vi "REPORT_PACE_prepare_header_for_pdf.vi"(11 "REPORT_PACE_all_info":T1) -> (3 "report_header":string[][](array[string]))   [LabVIEW 2019]
uses:
  typedef/REPORT_PACE_all_info.ctl
  _misc/AULocalize/SubVIs/Get Localized Phrase Compact Interface 1D.vi
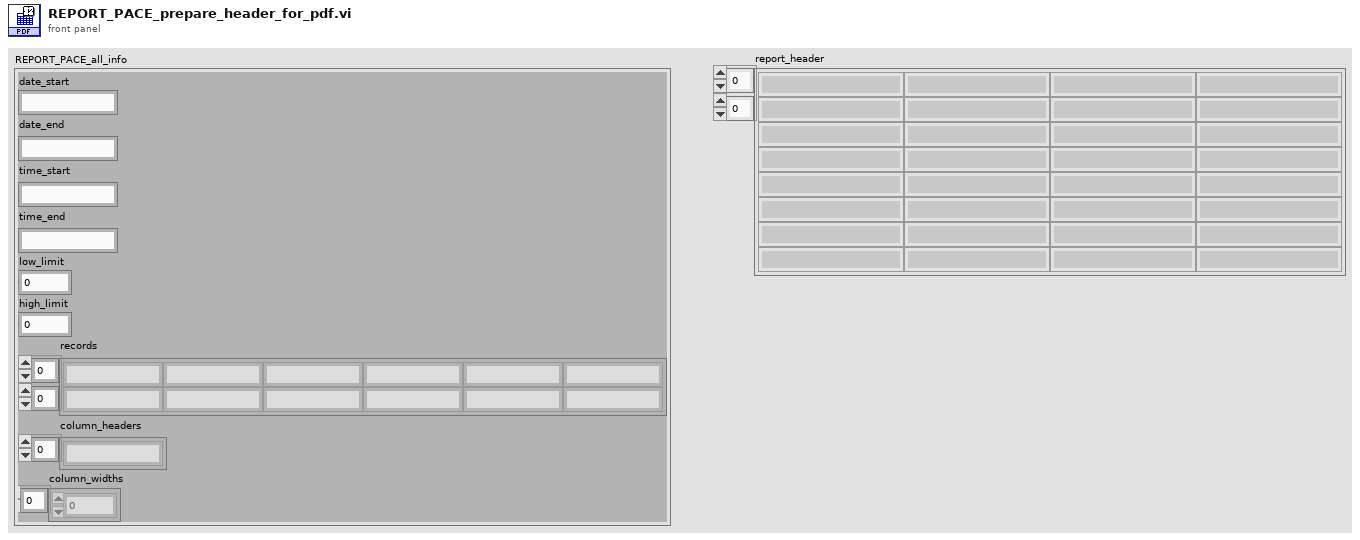
[diagram p1: front panel]
types:
  T1 = typedef "REPORT_PACE_all_info.ctl" = cluster{"date_start":string, "date_end":string, "time_start":string, "time_end":string, "low_limit":u16, "high_limit":u16, "records":string[][], "column_headers":string[], "column_widths":i16[]}
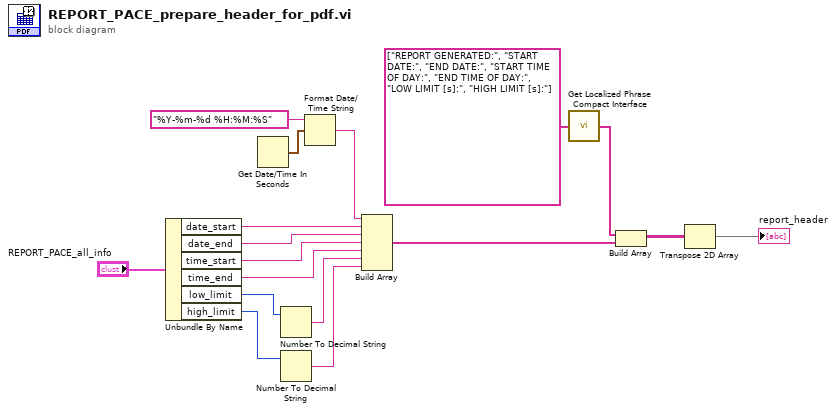
[diagram p0: block diagram]
diagram:
  n1 = Unbundle By Name("REPORT_PACE_all_info") -> ("date_start"=w9:string, "date_end"=w8:string, "time_start"=w7:string, "time_end"=w6:string, "low_limit"=w5:u16, "high_limit"=w3:u16)
  n2 = Get Date/Time In Seconds() -> (seconds since 1Jan1904=w16:timestamp)
  n3 = Number To Decimal String(number=w5) -> (decimal integer string=w4:string)  [unwired: 1 in]
  n4 = Number To Decimal String(number=w3) -> (decimal integer string=w2:string)  [unwired: 1 in]
  n5 = Format Date/Time String(time format string (%c)="%Y-%m-%d %H:%M:%S", seconds (now)=w16) -> (date/time string=w10:string)  [unwired: 1 in]
  n6 = Build Array(w10, w9, w8, w7, w6, w4, w2) -> (w11:string[])
  n7 = call-poly "Get Localized Phrase Compact Interface.vi"("Key"=string[] ["REPORT GENERATED:", "START DATE:", "END DATE:", "START TIME OF DAY:", "END TIME OF DAY:", "LOW LIMIT [s]:", "HIGH LIMIT [s]:"]) -> ("Translated Phrase"=w1:string[])
  n8 = Build Array(w1, w11) -> (w14:string[][])
  n9 = Transpose 2D Array(2D array=w14) -> (transposed array=→"report_header":string[][])
